vi "String To 2D String.vi"(7 "Delimiter":string=",", 10 "String In":string) -> (2 "2D String Out":string[][](array[string]))   [LabVIEW 2024]
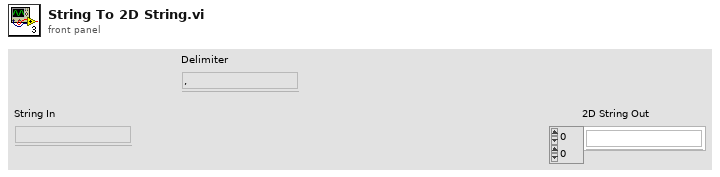
[diagram p1: front panel]
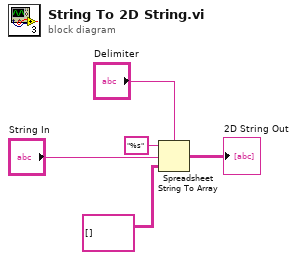
[diagram p0: block diagram]
diagram:
  n1 = Spreadsheet String To Array(delimiter (Tab)="Delimiter", format string="%s", spreadsheet string="String In", array type (2D Dbl)=string[][] []) -> (array=→"2D String Out":string[][])
